vi "Basic Then Callback.vi"(8 "error in (no error)":errorcluster, 9 "Scope":variant, 11 "Value":variant) -> (0 "error out":errorcluster)   [LabVIEW 2017, in "Unit Tests.lvlib"]
uses:
  Unit Tests.lvlib
  d6c984a8-2013-4802-b4e4-a7e52877237f.vi
  Promise Future/Promise/Promise.lvclass
  E:/Promise/Promise/Future/Future.lvclass
  Promise Future/Future/Fulfull (Value).vi
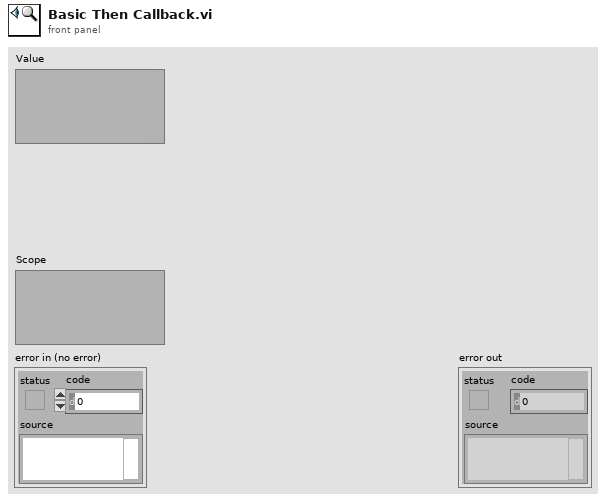
[diagram p1: front panel]
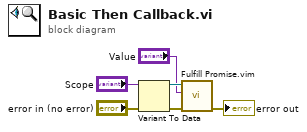
[diagram p0: block diagram]
diagram:
  n1 = Variant To Data(error in="error in (no error)", Variant="Scope") -> (data=w4:refnum<class "Promise.lvclass">, error out=w2:errorcluster)  [unwired: 1 in]
  n2 = call "Fulfill Promise.vim"("error in (no error)"=w2, "Value"="Value", "Promise in"=w4) -> ("error out"=→"error out":errorcluster)  [unwired: 7 in, 1 out]
